vi "PXI-Find DO Lines.vi"(11 "error in (no error)":errorcluster) -> (4 "DO.Lines":tag[](array[tag]), 15 "error out":errorcluster)   [LabVIEW 2015]
uses:
  <resource>/objmgr/daqmx.rc
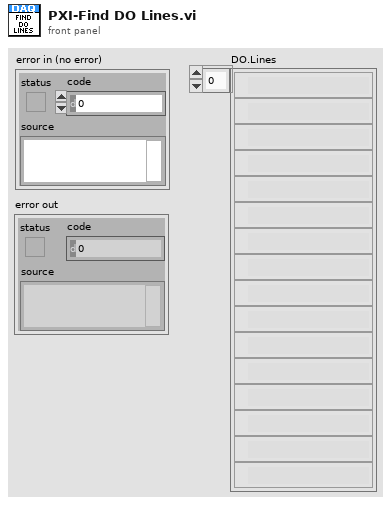
[diagram p1: front panel]
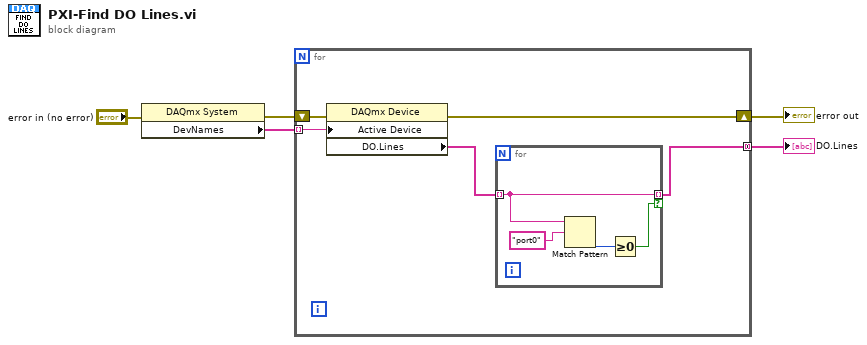
[diagram p0: block diagram]
diagram:
  n1 = property class="DAQmx System"(error in="error in (no error)") -> (error out=w3:errorcluster, "DevNames"=w4:tag[])  [unwired: 1 in, 1 out]
  n2 = for {
    tunnel: w4 -> [w9] mode=indexing
    shift-right: [w10] -> w2
    shift-left: w3 -> [w8]
    tunnel: [w6] -> w1 mode=concatenating
    n3 = property class="DAQmx Device"(error in=w8, "Active Device"=w9) -> (error out=w10:errorcluster, "DO.Lines"=w7:tag[])  [unwired: 1 in, 1 out]
    n4 = for {
      tunnel: w7 -> [w13] mode=indexing
      tunnel: [w13] -> w6 mode=indexing if=w11
      n5 = Match Pattern(string=w13, regular expression="port0") -> (offset past match=w12:i32)  [unwired: 1 in, 3 out]
      n6 = Greater Or Equal To 0?(x=w12) -> (x >= 0?=w11:bool)
    }
  }
  "error out" <- w2
  "DO.Lines" <- w1
